vi "Case.vi"(8 "Enum":enum16{"add", "sub", "mul", "div"}(ring), 10 "B":dbl, 11 "A":dbl) -> (3 "ans":dbl)   [LabVIEW 2020]
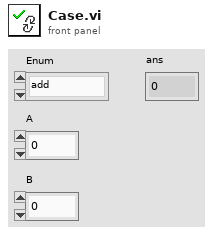
[diagram p1: front panel]
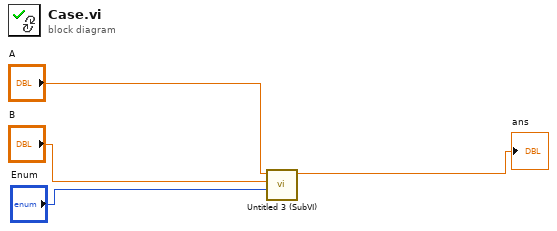
[diagram p0: block diagram]
diagram:
  n1 = call "Untitled 3 (SubVI).vi"("Enum"="Enum", "B"="B", "A"="A") -> ("Numeric"=→"ans":dbl)  [unwired: 8 in]
